vi "Controlling Timing.vi"(1 "Time":dbl) -> (0 "New Time":dbl)   [LabVIEW 2019]
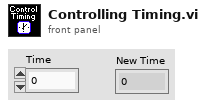
[diagram p1: front panel]
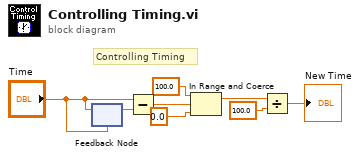
[diagram p0: block diagram]
diagram:
  # "Controlling Timing"
  n1 = feedback #1("Time") -> (w8:dbl)
  n2 = feedback-in #1("Time") -> ()
  n3 = Subtract(x="Time", y=w8) -> (x-y=w5:dbl)
  n4 = In Range and Coerce(upper limit=100.0, x=w5, lower limit=0.0) -> (coerced(x)=w4:dbl)  [unwired: 1 out]
  n5 = Divide(x=w4, y=100.0) -> (x/y=→"New Time":dbl)
